vi "Test Generated Mock Class Creates When VIs.vi"(8 "error in (no error)":errorcluster, 11 "Test Case In":refnum<class "Responsive Mock Class Generator Test.lvclass">) -> (0 "error out":errorcluster, 3 "Test Case Out":refnum<class "Responsive Mock Class Generator Test.lvclass">)   [LabVIEW 2020, in "Responsive Mock Class Generator Test.lvclass"]
uses:
  Responsive Mock Class Generator Test.lvclass
  C:/Program Files (x86)/National Instruments/LabVIEW 2020/vi.lib/Astemes/LUnit/Test Case.lvclass
  <vilib>/Astemes/LUnit/Test Case.lvclass/Test Case.ctl
  <vilib>/Astemes/LUnit/Append Fail Result.vi
  <vilib>/Astemes/LUnit/Append Pass Result.vi
  Responsive Mock Class Generator Test.lvclass/Responsive Mock Class Generator Test.ctl
  source/Scripting/Mock Class Generator/Responsive Mock Class Generator.lvclass
  source/Scripting/Interface Identifier/Interface Identifier.lvclass
  <vilib>/Astemes/LUnit/Test Case.lvclass
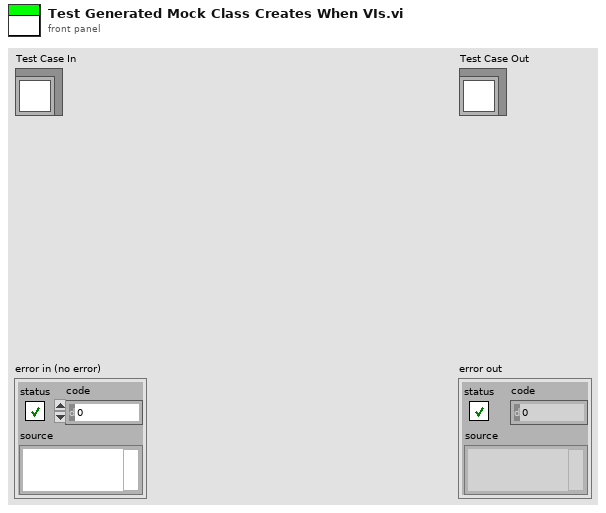
[diagram p1: front panel]
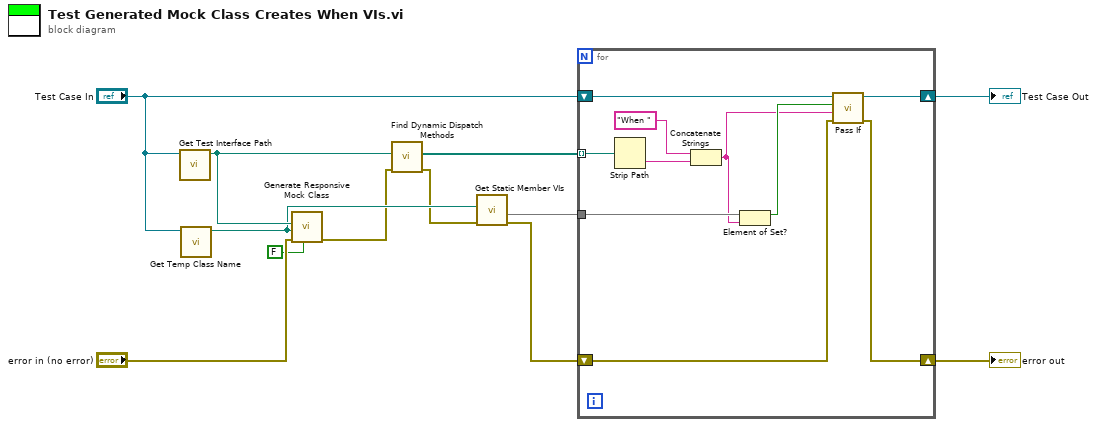
[diagram p0: block diagram]
diagram:
  n1 = call "Get Test Interface Path.vi"("Mock Class Generator Test in"="Test Case In") -> ("Test Class Path"=w8:path)  [unwired: 10 in]
  n2 = call "Get Temp Class Name.vi"("Mock Class Generator Test in"="Test Case In") -> ("Test Class Path"=w7:path)  [unwired: 10 in]
  n3 = call "Generate Responsive Mock Class.vi"("Add to lvproj?"=FALSE, "error in (no error)"="error in (no error)", "Destination Class Path"=w7, "Source Class Path"=w8) -> ("error out"=w5:errorcluster)  [unwired: 7 in]
  n4 = call "Find Dynamic Dispatch Methods.vi"("error in (no error)"=w5, "Class Path"=w8) -> ("error out"=w6:errorcluster, "Dynamic Dispatch VIs"=w2:path[])  [unwired: 8 in]
  n5 = call "Get Static Member VIs.vi"("error in (no error)"=w6, "Test Class Path"=w7) -> ("error out"=w4:errorcluster, "VI Names"=w1:set{string})  [unwired: 7 in, 1 out]
  n6 = for {
    shift-right: [w22] -> w12
    shift-left: "Test Case In" -> [w20]
    shift-right: [w21] -> w11
    shift-left: w4 -> [w19]
    tunnel: w2 -> [w18] mode=indexing
    tunnel: w1 -> [w15]
    n7 = Strip Path(path=w18) -> (name=w17:string)  [unwired: 1 out]
    n8 = Concatenate Strings("When " ("string"), w17) -> (w13:string)
    n9 = Element of Set?(10:w13, 11:w15) -> (3:w14:bool)
    n10 = call <vilib>:"Pass If.vi"("error in (no error)"=w19, "Message"=w13, "Pass?"=w14, "LUnit Test Case In"=w20) -> ("error out"=w21:errorcluster, "LUnit Test Case Out"=w22:refnum<class "Responsive Mock Class Generator Test.lvclass">)  [unwired: 6 in]
  }
  "error out" <- w11
  "Test Case Out" <- w12
